vi "Vbias dB To Word.vi"(0 "dB":dbl) -> (4 "Vbias Word":u8 format="%08b")   [LabVIEW 2020]
uses:
  <vilib>/gmath/NI_Gmath.lvlib
  9b3954db-bb76-4350-b219-fa9f862701d0.vi
panel:
  in  "Vbias 14.1V":u8=255 format="%08b"
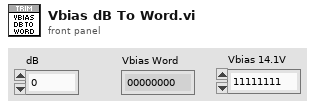
[diagram p1: front panel]
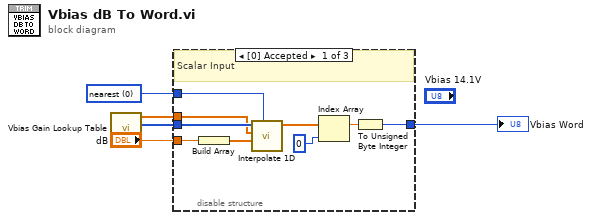
[diagram p0: block diagram]
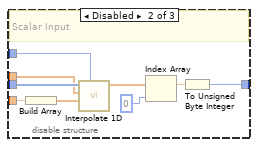
[diagram p2: hidden frame]
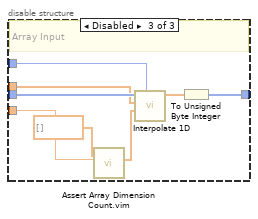
[diagram p3: hidden frame]
diagram:
  w5 = 0 items=["nearest", "linear", "spline", "cubic Hermite", "Lagrange"] ("method")
  n1 = call "Vbias Gain Lookup Table.vi"() -> ("ROUT<7:5>"=w4:u8[], "VB Gain(dB)"=w3:dbl[])  [unwired: 10 in]
  n2 = disable-structure shown="[0] Accepted" {
    disable-tunnel: w5 -> [w14 w23 w31]
    disable-tunnel: w4 -> [w13 w22 w30]
    disable-tunnel: w3 -> [w11 w20 w28]
    disable-tunnel: [w10 w19 w27] -> w1
    disable-tunnel: "dB" -> [w9 w18 w25]
    frame Enabled {
      # "Scalar Input"
      n3 = Build Array(w9) -> (w8:dbl[])
      n4 = call <vilib>:"Interpolate 1D.vi"("method"=w14, "xi"=w8, "X"=w11, "Y"=w13) -> ("yi"=w12:dbl[])  [unwired: 5 in, 2 out]
      n5 = Index Array(array=w12, index=0) -> (element=w7:dbl)
      n6 = To Unsigned Byte Integer(number=w7) -> (unsigned 8bit integer=w10:u8)
    }
    frame Disabled {
      # "Scalar Input"
      n7 = Build Array(w18) -> (w17:dbl[])
      n8 = call <vilib>:"Interpolate 1D.vi"("method"=w23, "xi"=w17, "X"=w20, "Y"=w22) -> ("yi"=w21:dbl[])  [unwired: 5 in, 2 out]
      n9 = Index Array(array=w21, index=0) -> (element=w16:dbl)
      n10 = To Unsigned Byte Integer(number=w16) -> (unsigned 8bit integer=w19:u8)
    }
    frame Disabled {
      # "Array Input"
      n11 = call "Assert Array Dimension Count.vim"("array type"=dbl[] [], "value in"=w25) -> ("value out"=w24:dbl[])  [unwired: 7 in]
      n12 = call <vilib>:"Interpolate 1D.vi"("method"=w31, "xi"=w24, "X"=w28, "Y"=w30) -> ("yi"=w29:dbl[])  [unwired: 5 in, 2 out]
      n13 = To Unsigned Byte Integer(number=w29) -> (unsigned 8bit integer=w27:u8[])
    }
  }
  "Vbias Word" <- w1
